vi "Initialize.vi"(8 "error in (no error)":errorcluster, 10 "DeviceName":string, 11 "FakePressureController in":refnum<class "DaqPad_NI6009.lvclass">) -> (0 "error out":errorcluster, 1 "new command(s)":string, 2 "DeviceName":string, 3 "FakePressureController out":refnum<class "DaqPad_NI6009.lvclass">)   [LabVIEW 2011, in "DaqPad_NI6009.lvclass"]
uses:
  DaqPad_NI6009.lvclass
  settings_TypDef.ctl
  OnOffTypeDef.ctl
  numericVariable_TypeDef.ctl
  BaseDriver/BaseDriver.lvclass
  DaqPad_NI6009.lvclass/DaqPad_NI6009.ctl
panel:
  out "variables to set":string[](array[string])
  out "numbers of channels":dbl
  out "DeviceName 2":string
  out "data":T1
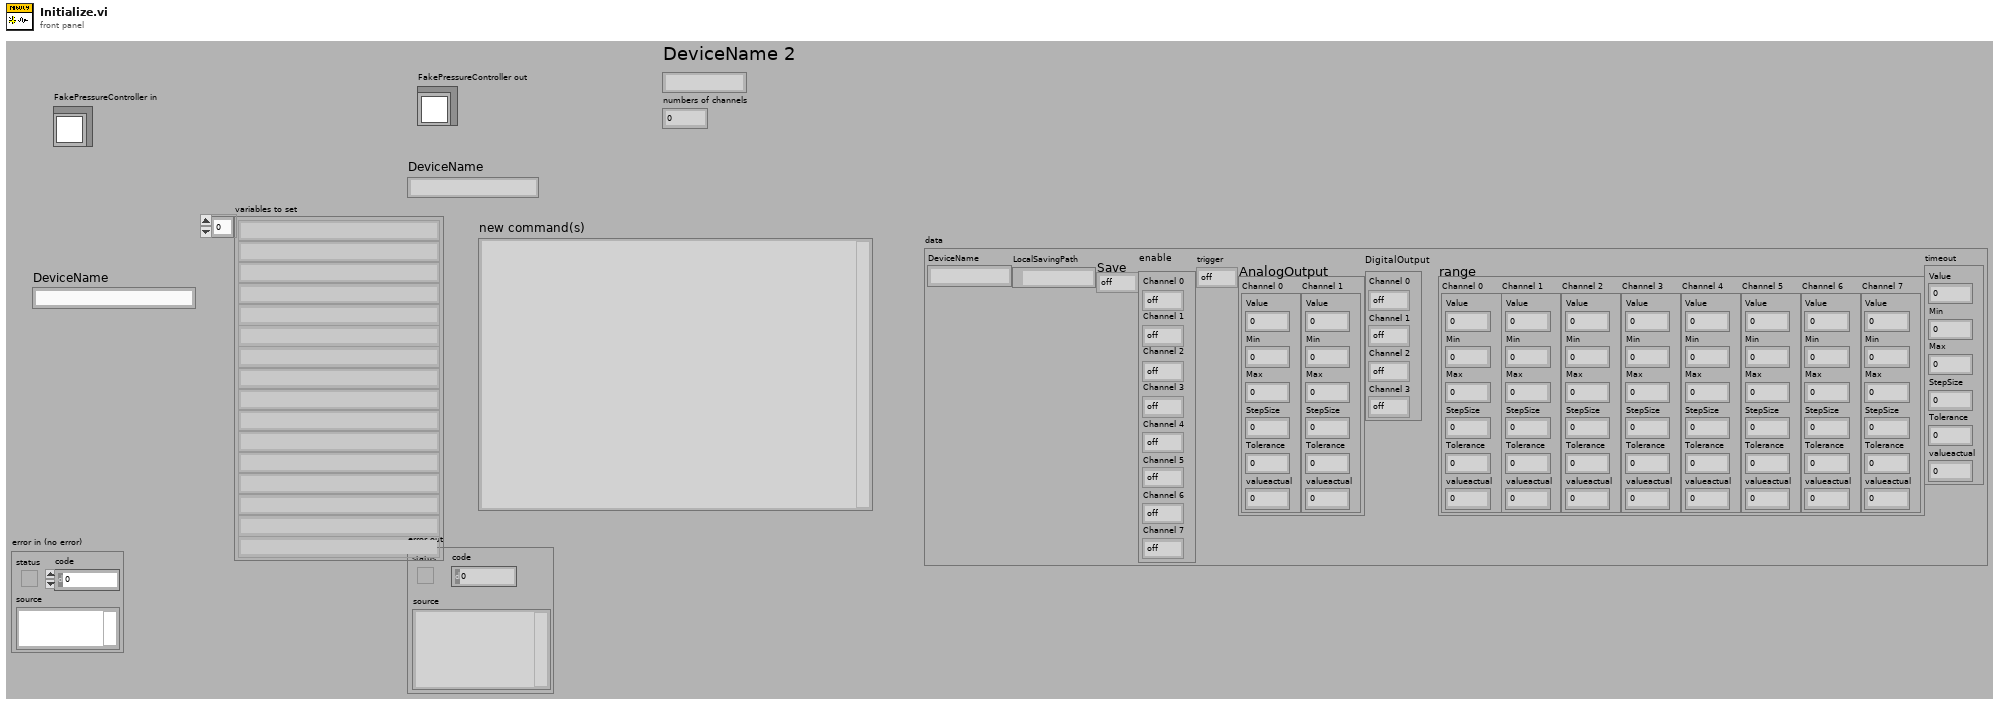
[diagram p1: front panel]
types:
  T1 = typedef "DaqPad_NI6009.lvclass/settings_TypDef.ctl" = cluster{"DeviceName":string, "LocalSavingPath":path, "Save":T2, "enable":cluster{"Channel 0":T2, "Channel 1":T2, "Channel 2":T2, "Channel 3":T2, "Channel 4":T2, "Channel 5":T2, "Channel 6":T2, "Channel 7":T2}, "trigger":T2, "AnalogOutput":cluster{"Channel 0":T3, "Channel 1":T3}, "DigitalOutput":cluster{"Channel 0":T2, "Channel 1":T2, "Channel 2":T2, "Channel 3":T2}, "range":cluster{"Channel 0":T3, "Channel 1":T3, "Channel 2":T3, "Channel 3":T3, "Channel 4":T3, "Channel 5":T3, "Channel 6":T3, "Channel 7":T3}, "timeout":T3}
  T2 = typedef "OnOffTypeDef.ctl" = enum16{"off", "on"}
  T3 = typedef "numericVariable_TypeDef.ctl" = cluster{"Value":dbl, "Min":dbl, "Max":dbl, "StepSize":dbl, "Tolerance":dbl, "valueactual":dbl}
  T4 = cluster{"Channel 0":T3, "Channel 1":T3, "Channel 2":T3, "Channel 3":T3, "Channel 4":T3, "Channel 5":T3, "Channel 6":T3, "Channel 7":T3}
  T5 = cluster{"Channel 0":T2, "Channel 1":T2, "Channel 2":T2, "Channel 3":T2, "Channel 4":T2, "Channel 5":T2, "Channel 6":T2, "Channel 7":T2}
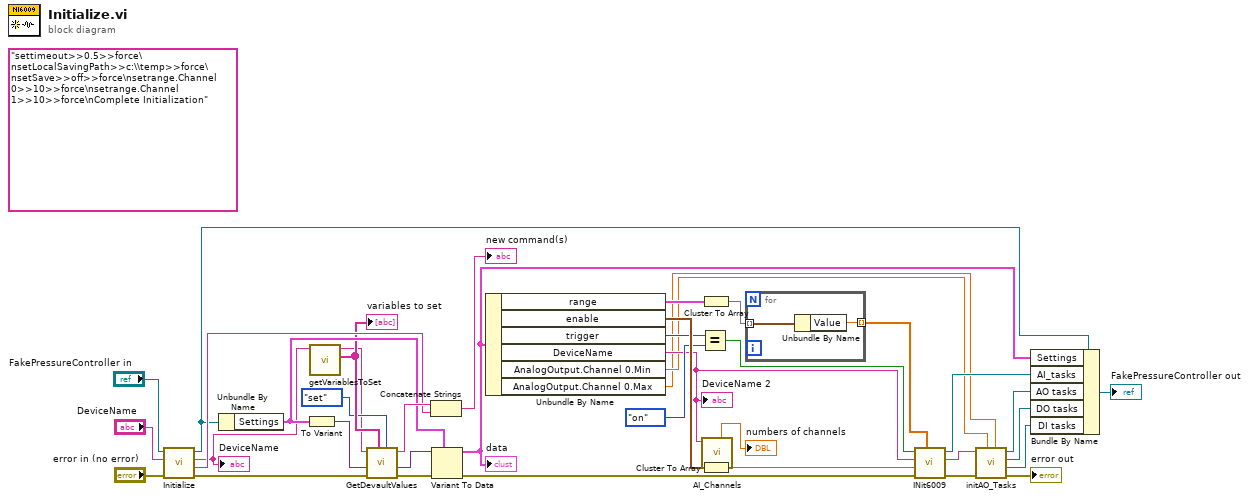
[diagram p0: block diagram]
diagram:
  (unwired) "settimeout>>0.5>>force\nsetLocalSavingPath>>c:\\temp>>force\nsetSave>>off>>force\nsetrange.Channel 0>>10>>force\nsetrange.Channel 1>>10>>force\nComplete Initialization" ("new command(s) 2")
  n1 = call-parent "Initialize.vi"("error in (no error)"="error in (no error)", "DeviceName"="DeviceName", "BaseDriver in"="FakePressureController in") -> ("error out"=w28:errorcluster, "new command(s)"=w31:string, "DeviceName"=w4:string, "BaseDriver out"=w30:refnum<class "DaqPad_NI6009.lvclass">)  [unwired: 5 in]
  "DeviceName" <- w4
  n2 = Unbundle By Name(w30) -> ("Settings"=w32:T1)
  n3 = To Variant(anything=w32) -> (Variant=w33:variant)
  n4 = call "getVariablesToSet.vi"("ActiveDev in"=w4) -> ("variables to set"=w6:string[], "ActiveDev out"=w3:string)  [unwired: 9 in]
  "variables to set" <- w6
  n5 = call "GetDevaultValues.vi"("set or DON'T set"=enum16{"set", "DON'T set"}."set", "set following Variables (empty = all avriables)"=w6, "error in (no error)"=w28, "variant"=w33, "Device Name"=w3) -> ("error out"=w27:errorcluster, "variant out"=w34:variant, "new command(s)"=w35:string)  [unwired: 4 in]
  n6 = Concatenate Strings(w35, w31) -> (→"new command(s)":string)
  n7 = Variant To Data(error in=w27, type=w32, Variant=w34) -> (data=w26:T1, error out=w25:errorcluster)
  "data" <- w26
  n8 = Unbundle By Name(w26) -> ("range"=w24:T4, "enable"=w23:T5, "trigger"=w21:T2, "DeviceName"=w9:string, "AnalogOutput.Channel 0.Min"=w2:dbl, "AnalogOutput.Channel 0.Max"=w1:dbl)
  "DeviceName 2" <- w9
  n9 = Equal?(x=w21, y=OnOffTypeDef."on") -> (x = y?=w19:bool)
  n10 = Cluster To Array(cluster=w24) -> (array=w17:T3[])
  n11 = Cluster To Array(cluster=w23) -> (array=w22:T2[])
  n12 = call "AI_Channels.vi"("DAQmx Device Name"=w9) -> ("# AI"=→"numbers of channels":dbl)  [unwired: 9 in, 1 out]
  n13 = for {
    tunnel: w17 -> [w40] mode=indexing
    tunnel: [w39] -> w16 mode=indexing
    n14 = Unbundle By Name(w40) -> ("Value"=w39:dbl)
  }
  n15 = call "INit6009.vi"("Range"=w16, "error in (no error)"=w25, "ChannelEnable"=w22, "DAQmx Device Name"=w9, "Trigger"=w19) -> ("error out"=w14:errorcluster, "DAQmx Device Name out"=w13:tag, "Refnum out"=w18:refnum<k21>)  [unwired: 4 in]
  n16 = call "initAO_Tasks.vi"("maximum value"=w1, "minimum value"=w2, "error in (no error)"=w14, "DAQmx Device Name 2"=w13) -> ("error out"=→"error out":errorcluster, "DI tasks"=w10:refnum<k21>, "DO tasks"=w11:refnum<k21>, "AO tasks"=w12:refnum<k21>)  [unwired: 4 in]
  n17 = Bundle By Name(cluster=w30, "Settings"=w26, "AI_tasks"=w18, "AO tasks"=w12, "DO tasks"=w11, "DI tasks"=w10) -> (→"FakePressureController out":refnum<class "DaqPad_NI6009.lvclass">)
